vi "引用測試3.vi"() -> ()   [LabVIEW 2015]
uses:
  <vilib>/vision/Measure.llb/Edge Options.ctl
  <vilib>/vision/Measure.llb/Edge Polarity.ctl
  <vilib>/userdefined/High Color/IMAQdx.ctl
  <vilib>/vision/driver/NI_Vision_Acquisition_Software.lvlib
  <vilib>/vision/NI_Vision_Development_Module.lvlib
panel:
  in  "重新開圖":bool
  out "Line Data":cluster{"X":sgl, "Y":sgl, "T":sgl}
  in  "開圖":bool
  in  "ShowData":bool
  in  "DieArea":i32=100 min=10
  in  "動作":enum16{"什麼也不做", "抓邊", "看灰階", "分析光源均勻度"}(ring)
  out "Mean":sgl format="%#.2f"
  out "Histogram":T1(graph)
  in  "取像":bool
  in  "Edge Options":T2={"Edge Polarity"=0, "Kernel Size"=3, "Width"=3, "Minimum Edge Strength"=10.0, "Interpolation Type"=enum."Bilinear Fixed", "Data Processing Method"=enum."Average"} {"Edge Polarity" items=["All Edges", "Rising Edges", "Falling Edges"]; "Minimum Edge Strength" format="%.2f"; "Width" step=2; "Kernel Size" step=2}
  out "error out":errorcluster
  out "Ellipse":T4 {"Minor Axis"."Point 2"."Y" format="%.2f"; "Minor Axis"."Point 2"."X" format="%.2f"; "Minor Axis"."Point 1"."Y" format="%.2f"; "Minor Axis"."Point 1"."X" format="%.2f"; "Major Axis"."Point 2"."Y" format="%.2f"; "Major Axis"."Point 2"."X" format="%.2f"; "Major Axis"."Point 1"."Y" format="%.2f"; "Major Axis"."Point 1"."X" format="%.2f"; "Center"."Y" format="%.2f"; "Center"."X" format="%.2f"}
  in  "圓":enum16{"Inner to Outer", "Outer to Inner"}(ring)
  out "Gradient Information":dbl[][](graph)
  in  "邊":T5(ring)
  in  "Process":T6(ring)
  in  "Gap":i32=10 min=1 max=300
  in  "stop":bool
  out "Image":T7(plugin-control)
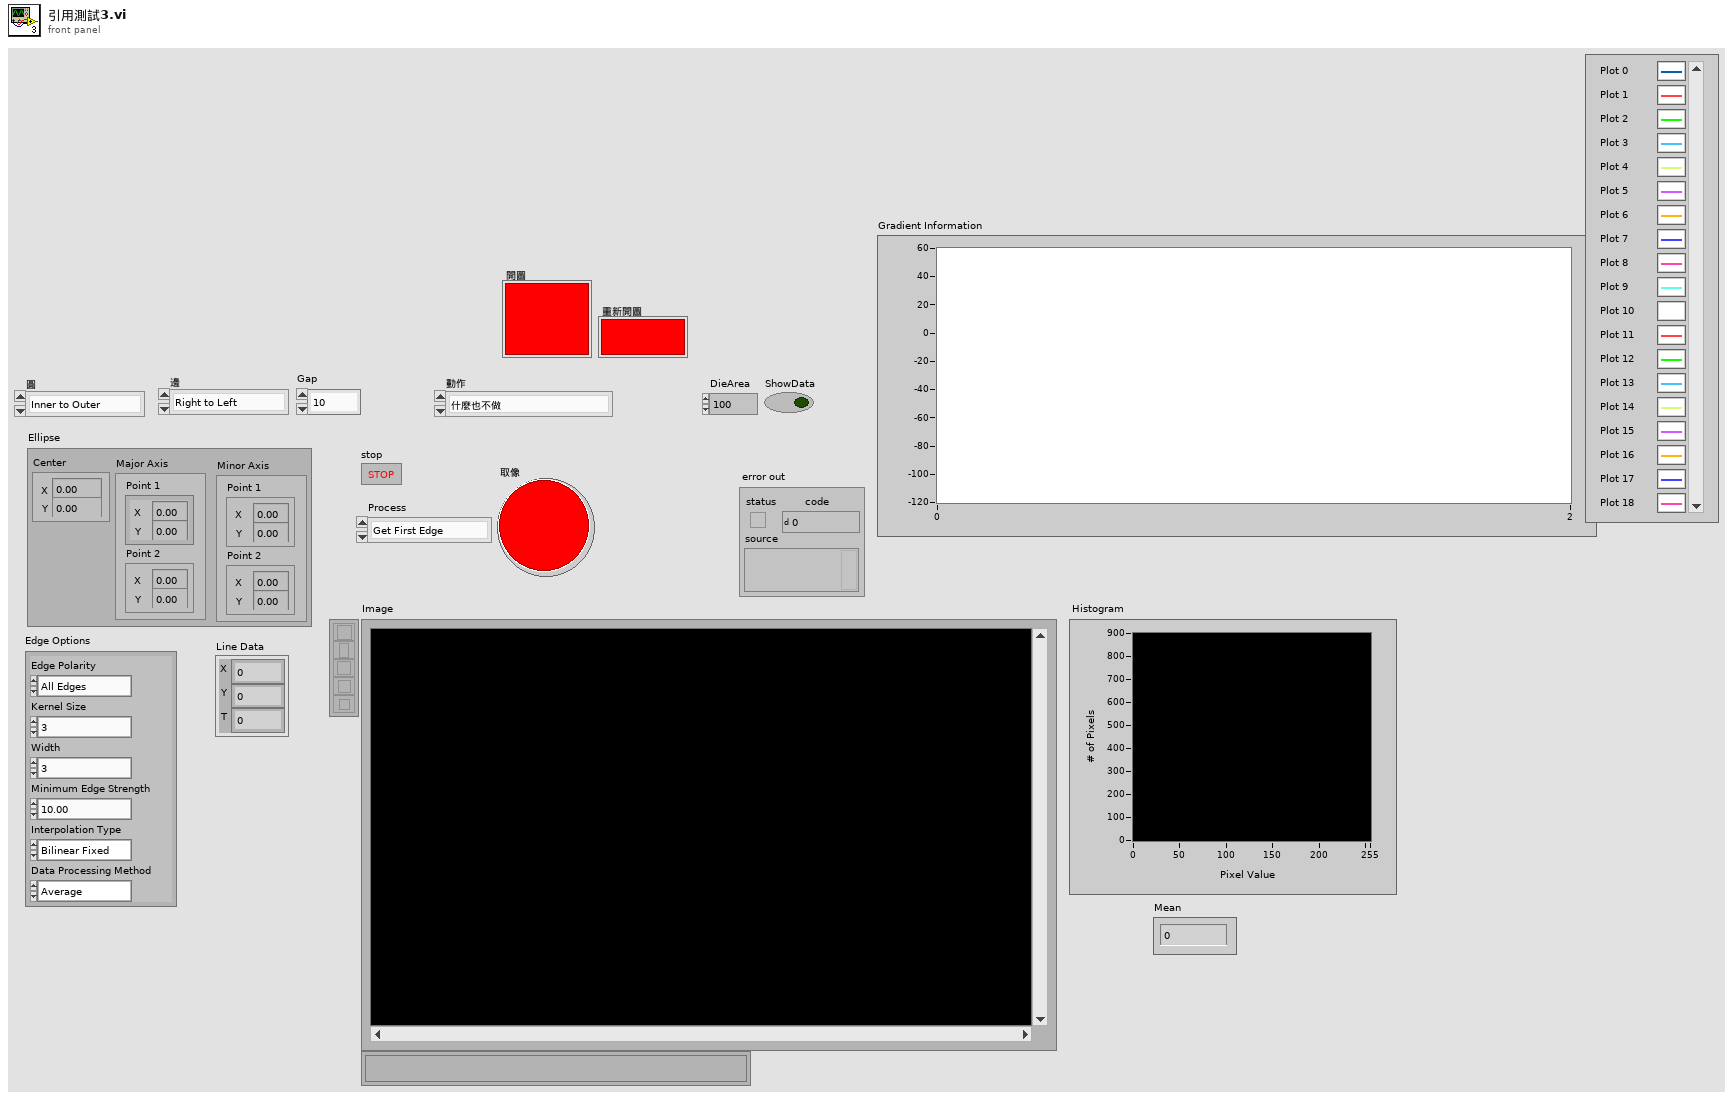
[diagram p1: front panel]
types:
  T1 = cluster{"Starting Value":sgl, "Incremental Value":sgl, "Histogram":u32[]}
  T2 = typedef "Edge Options.ctl" = cluster{"Edge Polarity":T3, "Kernel Size":u32, "Width":u32, "Minimum Edge Strength":sgl, "Interpolation Type":enum32{"Zero Order", "Bilinear", "Quadratic", "Cubic", "Bilinear Fixed"}, "Data Processing Method":enum32{"Average", "Median"}}
  T3 = typedef "Edge Polarity.ctl" = u32
  T4 = cluster{"Center":cluster{"X":sgl, "Y":sgl}, "Major Axis":cluster{"Point 1":cluster{"X":sgl, "Y":sgl}, "Point 2":cluster{"X":sgl, "Y":sgl}}, "Minor Axis":cluster{"Point 1":cluster{"X":sgl, "Y":sgl}, "Point 2":cluster{"X":sgl, "Y":sgl}}}
  T5 = enum16{"Right to Left", "Left  to Right", "Up to Down", "Down to Up"}
  T6 = enum16{"Get First Edge", "Get First + Last Edge", "Get All Edges", "Get Best Edge"}
  T7 = typedef "IMAQ Image.ctl" = refnum<image>
  T8 = typedef "IMAQ Rectangle" = cluster{"Left":i32, "Top":i32, "Right":i32, "Bottom":i32, "Rotation":dbl}
  T9 = typedef "IMAQdx.ctl" = refnum<k21>
  T10 = typedef "ROI Descriptor" = cluster{"Global Rectangle":i32[], "Contours":cluster{"ID":enum32{"External", "Internal"}, "Type":u32, "Coordinates":i32[]}[]}
  T11 = typedef "Image Type" = u32
  T12 = cluster{"Global Rectangle":i32[], "Contours":cluster{"Contour Type":u32, "ROI Type":u32, "Points":i32[]}[]}
  T13 = cluster{"Contour Type":u32, "ROI Type":u32, "Points":i32[]}[]
  T14 = cluster{"Contour Type":u32, "ROI Type":u32, "Points":i32[]}
  T15 = enum32{"Zero Order", "Bilinear", "Quadratic", "Cubic", "Bilinear Fixed"}
  T16 = cluster{"邊":enum16{"Right to Left", "Left  to Right", "Up to Down", "Down to Up"}, "動作":enum16{"什麼也不做", "抓邊", "看灰階", "分析光源均勻度"}, "圓":enum16{"Inner to Outer", "Outer to Inner"}, "Process":enum16{"Get First Edge", "Get First + Last Edge", "Get All Edges", "Get Best Edge"}, "ROI Type":u32, "Gap":i32, i32, i32, i32, i32, "Edge Polarity":T3, "Kernel Size":u32, "Width":u32, "Minimum Edge Strength":sgl, "Interpolation Type":enum32{"Zero Order", "Bilinear", "Quadratic", "Cubic", "Bilinear Fixed"}, "Data Processing Method":enum32{"Average", "Median"}, "DieArea":i32, "ShowData":bool}
  T17 = cluster{"邊":bool, "動作":bool, "圓":bool, "Process":bool, "ROI Type":bool, "Gap":bool, bool, bool, bool, bool, "Edge Polarity":bool, "Kernel Size":bool, "Width":bool, "Minimum Edge Strength":bool, "Interpolation Type":bool, "Data Processing Method":bool, "DieArea":bool, "ShowData":bool}
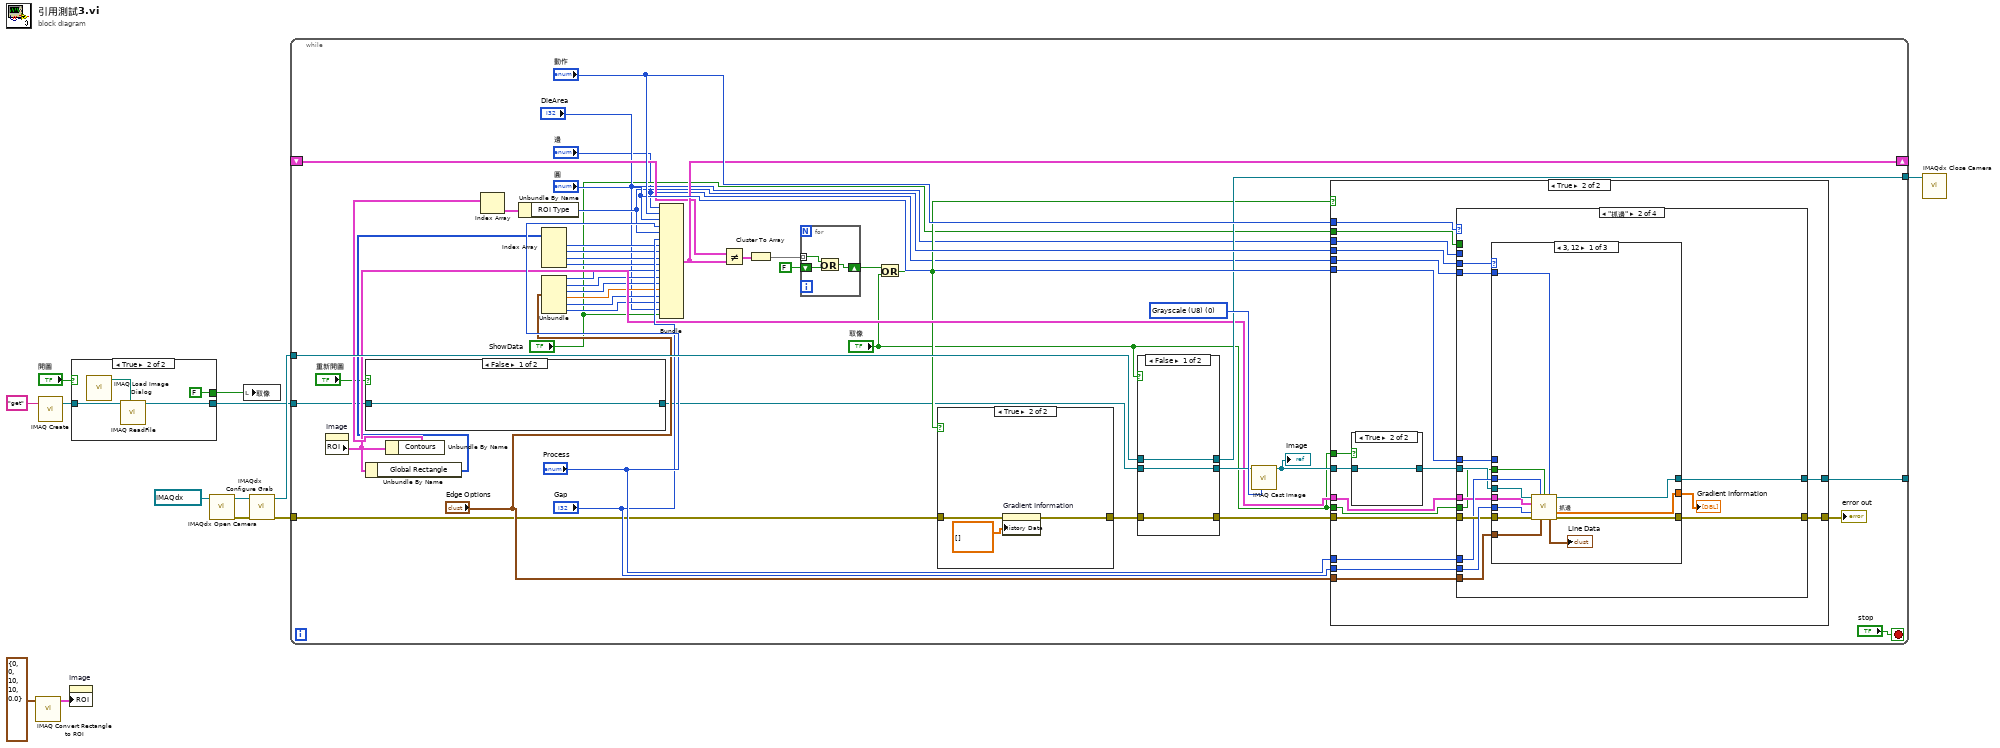
[diagram p0: block diagram]
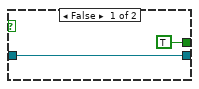
[diagram p2: hidden frame]
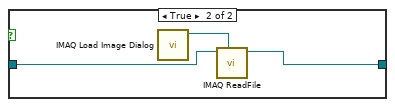
[diagram p3: hidden frame]
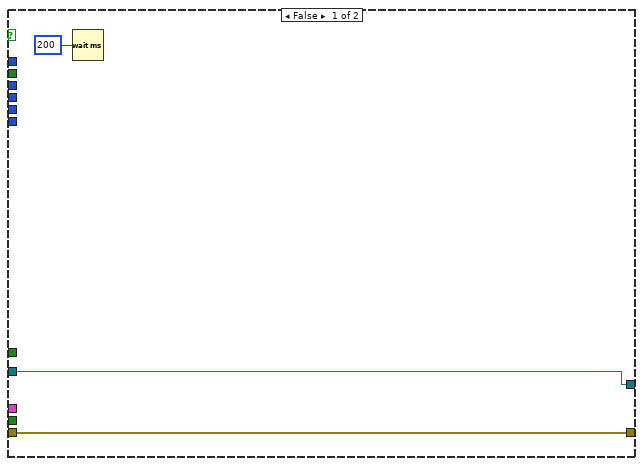
[diagram p5: hidden frame]
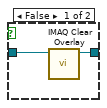
[diagram p6: hidden frame]
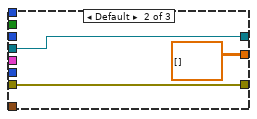
[diagram p8: hidden frame]
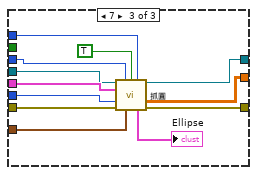
[diagram p9: hidden frame]
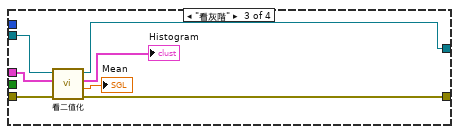
[diagram p10: hidden frame]
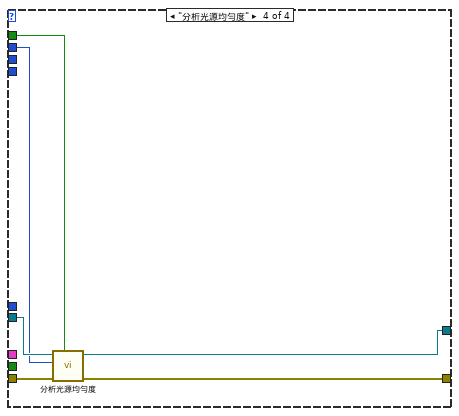
[diagram p11: hidden frame]
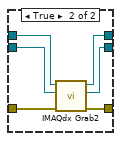
[diagram p12: hidden frame]
diagram:
  n1 = call "IMAQ Convert Rectangle to ROI"("Rectangle"=T8 {"Left"=0, "Top"=0, "Right"=10, "Bottom"=10, "Rotation"=0.0}) -> ("ROI Descriptor"=w6:T10)  [unwired: 8 in, 1 out]
  n2 = call "IMAQ Create"("Image Name"="get") -> ("New Image"=w3:T7)  [unwired: 4 in, 1 out]
  n3 = property on="Image" class="ImageControl"("ROI"=w6) -> ()  [unwired: 2 in, 2 out]
  n4 = case shown="True" "開圖" {
    tunnel: [TRUE ("取像") FALSE ("取像")] -> w4
    tunnel: w3 -> [w14 w18]
    tunnel: [w14 w17] -> w2
    frame False {
    }
    frame True {
      n5 = call "IMAQ Load Image Dialog"() -> ("Path"=w16:path)  [unwired: 9 in, 2 out]
      n6 = call "IMAQ ReadFile"("File Path"=w16, "Image"=w18) -> ("Image Out"=w17:T7)  [unwired: 5 in, 4 out]
    }
  }
  n7 = call <vilib>:"IMAQdx Open Camera.vi"("Session In"=T9 "cam1") -> ("error out"=w8:errorcluster, "Session Out"=w9:T9)  [unwired: 9 in]
  n8 = local write "取像"(w4) -> ()
  n9 = call <vilib>:"IMAQdx Configure Grab.vi"("error in"=w8, "Session In"=w9) -> ("error out"=w1:errorcluster, "Session Out"=w12:T9)  [unwired: 8 in]
  n10 = while {
    tunnel: w12 -> [w64]
    tunnel: w2 -> [w21]
    tunnel: [w44] -> w11
    tunnel: [w58] -> _
    shift-right: [w53] -> _
    shift-left: _ -> [w52]
    tunnel: w1 -> [w25]
    stop <- "stop" stop-if-true
    w62 = T11 0 items=["Grayscale (U8)", "Grayscale (I16)", "Grayscale (SGL)", "Complex (CSG)", "RGB (U32)", "HSL (U32)", "RGB (U64)", "Grayscale (U16)"] ("Image Type")
    n11 = property on="Image" class="ImageControl"() -> ("ROI"=w42:T12)  [unwired: 2 in, 2 out]
    n12 = case shown="False" "重新開圖" {
      tunnel: w21 -> [w65 w66]
      tunnel: [w65 w67] -> w20
      frame False {
      }
      frame True {
        n13 = call "IMAQ Load Image Dialog"() -> ("Path"=w68:path)  [unwired: 9 in, 2 out]
        n14 = call "IMAQ ReadFile"("File Path"=w68, "Image"=w66) -> ("Image Out"=w67:T7)  [unwired: 5 in, 4 out]
      }
    }
    n15 = Unbundle By Name(w42) -> ("Global Rectangle"=w41:i32[])
    n16 = Unbundle By Name(w42) -> ("Contours"=w57:T13)
    n17 = Index Array(array=w57) -> (element=w56:T14)  [unwired: 1 in]
    n18 = Unbundle By Name(w56) -> ("ROI Type"=w46:u32)
    n19 = Index Array(array=w41) -> (element #1=w40:i32, element #2=w39:i32, element #3=w38:i32, element #4=w37:i32)  [unwired: 4 in]
    n20 = Unbundle("Edge Options") -> ("Edge Polarity"=w34:T3, "Kernel Size"=w33:u32, "Width"=w32:u32, "Minimum Edge Strength"=w31:sgl, "Interpolation Type"=w30:T15, "Data Processing Method"=w29:enum32{"Average", "Median"})
    n21 = Bundle("邊"="邊", "動作"="動作", "圓"="圓", "Process"="Process", "ROI Type"=w46, "Gap"="Gap", w40, w39, w38, w37, "Edge Polarity"=w34, "Kernel Size"=w33, "Width"=w32, "Minimum Edge Strength"=w31, "Interpolation Type"=w30, "Data Processing Method"=w29, "DieArea"="DieArea", "ShowData"="ShowData") -> (w53:T16)  [unwired: 1 in]
    n22 = Not Equal?(x=w52, y=w53) -> (x != y?=w45:T17)
    n23 = Cluster To Array(cluster=w45) -> (array=w51:bool[])
    n24 = for {
      tunnel: w51 -> [w75] mode=indexing
      shift-right: [w74] -> w49
      shift-left: FALSE -> [w73]
      n25 = Or(x=w75, y=w73) -> (x .or. y?=w74:bool)
    }
    n26 = Or(x=w49, y="取像") -> (x .or. y?=w36:bool)
    n27 = case shown="True" w36 {
      tunnel: [w69 w71] -> w61
      tunnel: w25 -> [w69 w70]
      frame False {
      }
      frame True {
        n28 = property on="Gradient Information" class="WFChart (strict)"(error in=w70, "History Data"=dbl[][] []) -> (error out=w71:errorcluster)  [unwired: 1 in, 1 out]
      }
    }
    n29 = case shown="False" "取像" {
      tunnel: w64 -> [w156 w162]
      tunnel: w20 -> [w155 w161]
      tunnel: [w156 w160] -> w44
      tunnel: [w155 w159] -> w43
      tunnel: w61 -> [w154 w158]
      tunnel: [w154 w157] -> w60
      frame False {
      }
      frame True {
        n30 = call <vilib>:"IMAQdx Grab2.vi"("error in"=w158, "Image In"=w161, "Session In"=w162) -> ("error out"=w157:errorcluster, "Image Out"=w159:T7, "Session Out"=w160:T9)  [unwired: 5 in, 1 out]
      }
    }
    n31 = call "IMAQ Cast Image"("Image Type"=w62, "Image Src"=w43) -> ("Image Dst Out"=w59:T7)  [unwired: 8 in, 1 out]
    "Image" <- w59
    n32 = case shown="True" w36 {
      tunnel: "Gap" -> [_ w95]
      tunnel: w60 -> [w78 w94]
      tunnel: "Process" -> [_ w93]
      tunnel: w59 -> [w77 w84]
      tunnel: [w77 w92] -> w58
      tunnel: w42 -> [_ w91]
      tunnel: w46 -> [_ w90]
      tunnel: "Edge Options" -> [_ w89]
      tunnel: [w78 w88] -> w24
      tunnel: "動作" -> [_ w87]
      tunnel: "圓" -> [_ w86]
      tunnel: "取像" -> [_ w85]
      tunnel: "取像" -> [_ w82]
      tunnel: "DieArea" -> [_ w81]
      tunnel: "ShowData" -> [_ w80]
      tunnel: "邊" -> [_ w79]
      frame False {
        n33 = Wait (ms)(milliseconds to wait=u32 200) -> ()  [unwired: 1 out]
      }
      frame True {
        n34 = case shown="True" w85 {
          tunnel: w84 -> [w96 w98]
          tunnel: [w97 w98] -> w83
          frame False {
            n35 = call "IMAQ Clear Overlay"("Image"=w96) -> ("Image Out"=w97:T7)  [unwired: 9 in, 1 out]
          }
          frame True {
          }
        }
        n36 = case shown="\"抓邊\"" w87 {
          tunnel: w95 -> [_ w113 _ _]
          tunnel: w94 -> [w99 w112 w144 w149]
          tunnel: w86 -> [_ w111 _ _]
          tunnel: w93 -> [_ w110 _ _]
          tunnel: w83 -> [w100 w109 w146 w151]
          tunnel: [w100 w108 w147 w152] -> w92
          tunnel: w91 -> [_ w107 w145 _]
          tunnel: w90 -> [_ w106 _ _]
          tunnel: w89 -> [_ w105 _ _]
          tunnel: [w99 w103 w141 w153] -> w88
          tunnel: w82 -> [_ w102 _ _]
          tunnel: w81 -> [_ _ _ w150]
          tunnel: w80 -> [_ _ _ w148]
          tunnel: w79 -> [_ w101 _ _]
          frame "什麼也不做", Default {
          }
          frame "抓邊" {
            n37 = case shown="3, 12" w106 {
              tunnel: w107 -> [w124 _ w134]
              tunnel: w113 -> [w123 _ w135]
              tunnel: w112 -> [w122 w126 w136]
              tunnel: w111 -> [_ _ w131]
              tunnel: w110 -> [w117 _ w132]
              tunnel: [w120 dbl[][] [] ("Gradient Information") w139] -> w104
              tunnel: w109 -> [w125 w128 w133]
              tunnel: [w119 w128 w140] -> w108
              tunnel: [w121 w126 w129] -> w103
              tunnel: w105 -> [w118 _ w137]
              tunnel: w102 -> [w116 _ _]
              tunnel: w101 -> [w114 _ _]
              frame 3, 12 {
                n38 = call "抓邊.vi"("Image In"=w125, "Process"=w117, "Optimized Mode"=w116, "Direction"=w114, "ROI"=w124, "Gap"=w123, "error In"=w122, "Edge Options"=w118) -> ("Image Out"=w119:T7, "Gradient Information"=w120:dbl[][], "Line Data"=→"Line Data":cluster{"X":sgl, "Y":sgl, "T":sgl}, "error out"=w121:errorcluster)  [unwired: 3 in, 1 out]
              }
              frame Default {
              }
              frame 7 {
                n39 = call "抓圓.vi"("Image In"=w133, "Process"=w132, "Optimized Mode"=TRUE, "Direction"=w131, "ROI"=w134, "Gap"=w135, "error In"=w136, "Edge Options"=w137) -> ("Imag e Out"=w140:T7, "Gradient Information"=w139:dbl[][], "Ellipse"=→"Ellipse":T4, "error out"=w129:errorcluster)  [unwired: 3 in, 1 out]
              }
            }
            "Gradient Information" <- w104
          }
          frame "看灰階" {
            n40 = call "看二值化.vi"("error in (no error)"=w144, "ROI Descriptor"=w145, "Image In"=w146) -> ("error out"=w141:errorcluster, "Mean"=→"Mean":sgl, "Histogram"=→"Histogram":T1, "Image Out"=w147:T7)  [unwired: 4 in, 1 out]
          }
          frame "分析光源均勻度" {
            n41 = call "分析光源均勻度.vi"("ShowData"=w148, "error in (no error)"=w149, "DieArea"=w150, "Image In"=w151) -> ("error out"=w153:errorcluster, "Image"=w152:T7)  [unwired: 6 in]
          }
        }
      }
    }
    "error out" <- w24
  }
  n42 = call <vilib>:"IMAQdx Close Camera.vi"("Session In"=w11) -> ()  [unwired: 10 in, 1 out]
